vi "FFTBoost.vi"(7 "CompensationCoefficients":dbl[](array[numeric])=[1.0, 1.0, 0.0, 0.0, 0.0], 10 "mutedData":dbl[](array[numeric])=array[1605632 elements], 11 "SamplingFreq (for graph)":dbl=500.0) -> (2 "boostedData":dbl[](array[numeric]))   [LabVIEW 2011]
uses:
  <vilib>/Analysis/2dsp.llb/Real FFT.vi
  <vilib>/Analysis/2dsp.llb/Inverse Real FFT.vi
  <vilib>/Analysis/NI_AALPro.lvlib
panel:
  out "CallCount":dbl
  out "Waveform Graph":cluster{i32, dbl, dbl[]}[](graph)
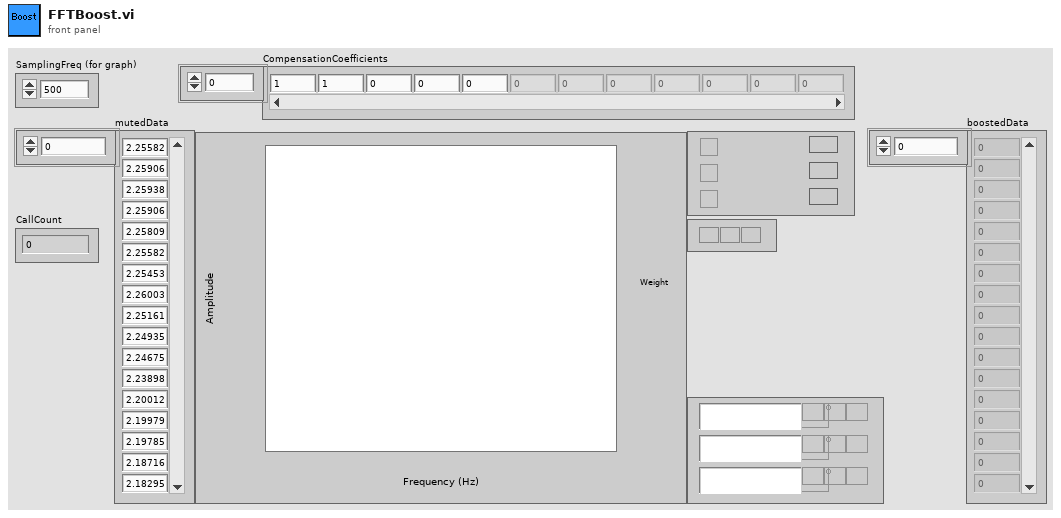
[diagram p1: front panel]
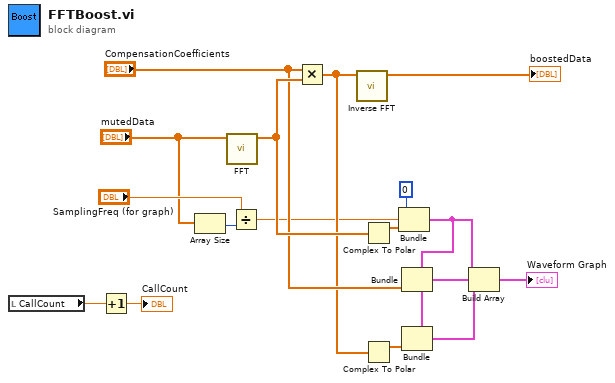
[diagram p0: block diagram]
diagram:
  n1 = local read "CallCount"() -> (w2:dbl)
  n2 = Increment(x=w2) -> (x+1=→"CallCount":dbl)
  n3 = Array Size(array="mutedData") -> (size(s)=w6:i32)
  n4 = call-poly <vilib>:"FFT.vi"("X"="mutedData") -> ("FFT {X}"=w16:cdb[])  [unwired: 2 in, 8 out]
  n5 = Divide(x="SamplingFreq (for graph)", y=w6) -> (x/y=w5:dbl)
  n6 = Multiply(x="CompensationCoefficients", y=w16) -> (x*y=w9:cdb[])
  n7 = call-poly <vilib>:"Inverse FFT.vi"("FFT {X}"=w9) -> ("X"=→"boostedData":dbl[])  [unwired: 1 in, 9 out]
  n8 = Complex To Polar(r * e^(i*theta)=w16) -> (r=w15:dbl[])  [unwired: 1 out]
  n9 = Complex To Polar(r * e^(i*theta)=w9) -> (r=w8:dbl[])  [unwired: 1 out]
  n10 = Bundle(0, w5, w15) -> (w12:cluster{i32, dbl, dbl[]})  [unwired: 1 in]
  n11 = Bundle(cluster=w12, "CompensationCoefficients") -> (w14:cluster{i32, dbl, dbl[]})  [unwired: 2 in]
  n12 = Bundle(cluster=w12, w8) -> (w13:cluster{i32, dbl, dbl[]})  [unwired: 2 in]
  n13 = Build Array(w12, w14, w13) -> (→"Waveform Graph":cluster{i32, dbl, dbl[]}[])
